vi "字符串查找.vi"() -> ()   [LabVIEW 2018]
panel:
  out "数组 3":i32[](array[numeric])
  out "字符串 2":string
  out "字符串":string
  out "数组 2":string[](array[string])
  out "数组":string[](array[string])
  out "匹配子字符串":string
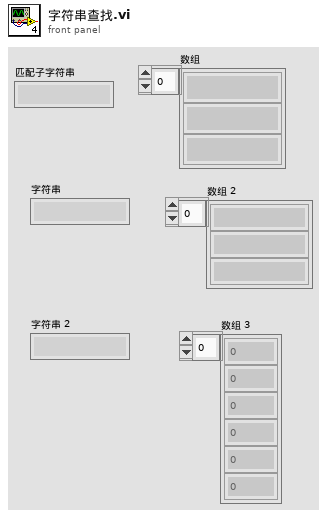
[diagram p1: front panel]
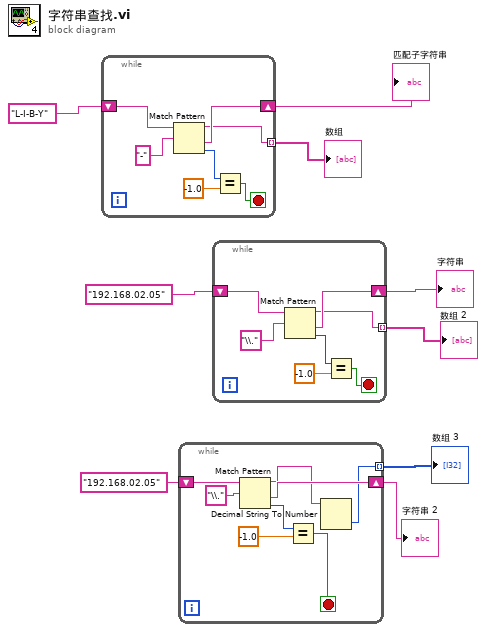
[diagram p0: block diagram]
diagram:
  n1 = while {
    tunnel: [w10] -> w7 mode=indexing
    shift-right: [w11] -> w8
    shift-left: "L-I-B-Y" ("字符串") -> [w16]
    stop <- w13 stop-if-true
    n2 = Match Pattern(string=w16, regular expression="-" ("正则表达式")) -> (before substring=w10:string, after substring=w11:string, offset past match=w12:i32)  [unwired: 1 in, 1 out]
    n3 = Equal?(x=w12, y=-1.0) -> (x = y?=w13:bool)
  }
  "匹配子字符串" <- w8
  "数组" <- w7
  n4 = while {
    tunnel: [w17] -> w1 mode=indexing
    shift-right: [w19] -> w2
    shift-left: "192.168.02.05" ("字符串") -> [w24]
    stop <- w21 stop-if-true
    n5 = Match Pattern(string=w24, regular expression="\\." ("正则表达式")) -> (before substring=w18:string, after substring=w19:string, offset past match=w20:i32)  [unwired: 1 in, 1 out]
    n6 = Equal?(x=w20, y=-1.0) -> (x = y?=w21:bool)
    n7 = Decimal String To Number(string=w18) -> (number=w17:i32)  [unwired: 2 in, 1 out]
  }
  "字符串 2" <- w2
  "数组 3" <- w1
  n8 = while {
    tunnel: [w25] -> w5 mode=indexing
    shift-right: [w26] -> w4
    shift-left: "192.168.02.05" ("字符串") -> [w31]
    stop <- w28 stop-if-true
    n9 = Match Pattern(string=w31, regular expression="\\." ("正则表达式")) -> (before substring=w25:string, after substring=w26:string, offset past match=w27:i32)  [unwired: 1 in, 1 out]
    n10 = Equal?(x=w27, y=-1.0) -> (x = y?=w28:bool)
  }
  "数组 2" <- w5
  "字符串" <- w4
